vi "BL_ConvertNumericIntoSingle.vi"(8 "error in (no error)":errorcluster, 9 "Number":i32, 11 "Potentiostat Galvanostat in":refnum<class "Potentiostat Galvanostat.lvclass">) -> (0 "error out":errorcluster, 1 "Single":sgl, 3 "Potentiostat Galvanostat out":refnum<class "Potentiostat Galvanostat.lvclass">)   [LabVIEW 2018, in "Potentiostat Galvanostat.lvclass"]
doc: "The hardware conf object. The attribute “Conn” is the electrode\nconnection mode and the attribute “Ground” is the instrument\nground. See 5. Structures and Constants to have the value of these\nattributes."
uses:
  Potentiostat Galvanostat.lvclass
  Potentiostat Galvanostat.lvclass/Potentiostat Galvanostat.ctl
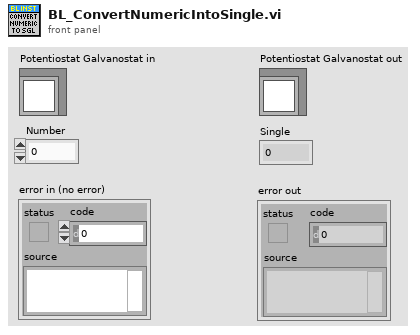
[diagram p1: front panel]
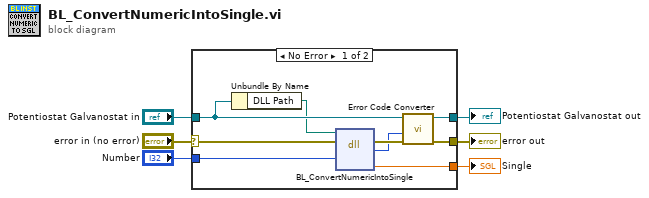
[diagram p0: block diagram]
diagram:
  n1 = case shown="No Error" "error in (no error)" {
    selector: "error in (no error)" -> [w12 w17]
    tunnel: [w15 w17] -> w5
    tunnel: [w14 w16] -> w3
    tunnel: "Potentiostat Galvanostat in" -> [w13 w16]
    tunnel: "Number" -> [w10 _]
    tunnel: [w7 _] -> w1
    frame No Error {
      n2 = Unbundle By Name(w13) -> ("DLL Path"=w11:path)
      n3 = dll-call lib="I:/Home Projects/LabVIEW/BioLogic Instrument Driver/libs/EC-Lab Development Package/EClib.dll" fn="BL_ConvertNumericIntoSingle" ("TI to IEEE")(path in=w11, error in=w12, "Number"=w10) -> (error out=w9:errorcluster, "Error Code"=w8:i32, "Single"=w7:sgl)  [unwired: 3 in, 1 out]
      n4 = call-dynamic "Error Code Converter.vi"("error in (no error)"=w9, "Error Code"=w8, "Potentiostat Galvanostat in"=w13) -> ("error out"=w15:errorcluster, "Potentiostat Galvanostat out"=w14:refnum<class "Potentiostat Galvanostat.lvclass">)  [unwired: 7 in]
    }
    frame Error {
    }
  }
  "error out" <- w5
  "Potentiostat Galvanostat out" <- w3
  "Single" <- w1
